vi "CRYLoad Operator Window Configure.vi"(8 "error in":errorcluster, 11 "File path":path) -> (0 "error out":errorcluster, 1 "ok status":bool, 2 "Flatten Step":string, 3 "selected path":path)   [LabVIEW 2013]
uses:
  CRYMainGlobal.vi
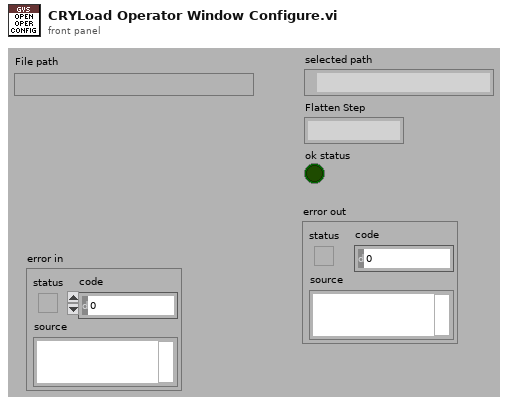
[diagram p1: front panel]
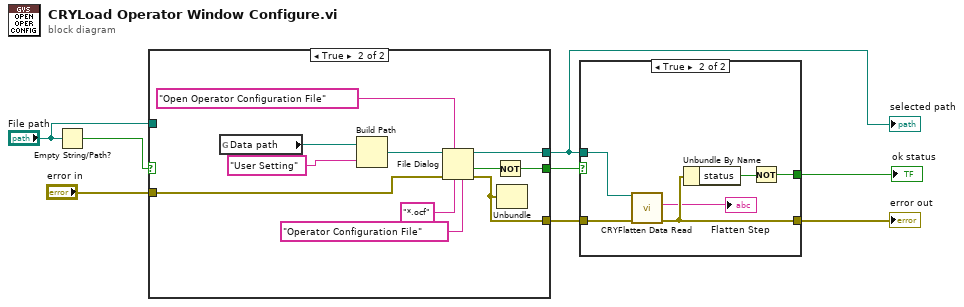
[diagram p0: block diagram]
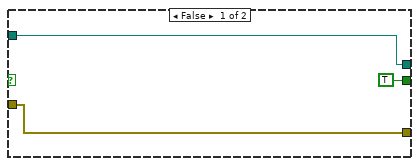
[diagram p2: hidden frame]
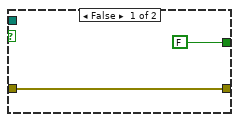
[diagram p3: hidden frame]
diagram:
  n1 = Empty String/Path?(string/path="File path") -> (empty?=w2:bool)
  n2 = case shown="True" w2 {
    tunnel: "error in" -> [w11 w21]
    tunnel: [TRUE w19] -> w7
    tunnel: [w10 w18] -> w5
    tunnel: [w11 w12] -> w4
    tunnel: "File path" -> [w10 _]
    frame False {
    }
    frame True {
      n3 = global read "CRYMainGlobal.vi" "Data path"() -> (w15:path)
      n4 = Build Path(base path=w15, name or relative path="User Setting") -> (appended path=w14:path)
      n5 = File Dialog(4:"Operator Configuration File" ("pattern label"), 6:"*.ocf" ("pattern (all files)"), 7:"Open Operator Configuration File", 8:w21, 11:w14) -> (0:w12:errorcluster, 1:w20:bool, 3:w18:path)  [unwired: 3 out]
      n6 = Not(x=w20) -> (.not. x?=w19:bool)
      n7 = Unbundle(w12) -> ()  [unwired: 3 out]
    }
  }
  "selected path" <- w5
  n8 = case shown="True" w7 {
    tunnel: w5 -> [_ w29]
    tunnel: [FALSE ("status") w25] -> w6
    tunnel: [w23 w27] -> w3
    tunnel: w4 -> [w23 w28]
    frame False {
    }
    frame True {
      n9 = call "CRYFlatten Data Read.vi"("error in"=w28, "Path In"=w29) -> ("error out"=w27:errorcluster, "Flatten Data Out"=→"Flatten Step":string)  [unwired: 5 in, 1 out]
      n10 = Unbundle By Name(w27) -> ("status"=w30:bool)
      n11 = Not(x=w30) -> (.not. x?=w25:bool)
    }
  }
  "ok status" <- w6
  "error out" <- w3
